vi "SV Get By Measurement Type (voltage) (N Ch).vi"(0 "scaled signals [EU]":waveform(dbl)[](array[waveform])) -> (4 "scaled signals with voltage channels deleted":waveform(dbl)[](array[waveform]), 6 "number of voltage channels":i32, 8 "voltage channels [V]":waveform(dbl)[](array[waveform]))   [LabVIEW 2017]
doc: "Separates data from an array of waveforms based on the type of measurement selected. This VI requires that waveform attributes such as NI_UnitDescription are added by NI DAQmx."
uses:
  <vilib>/addons/_NISVFA/_Shared subVIs/Groups/SV Match Unit.vi
  <vilib>/addons/_NISVFA/_Shared subVIs/Common/sv_Get NI Property Name String.vi
  <vilib>/addons/_NISVFA/_Shared subVIs/Groups/sv_ConcatenateArrayIndicies.vi
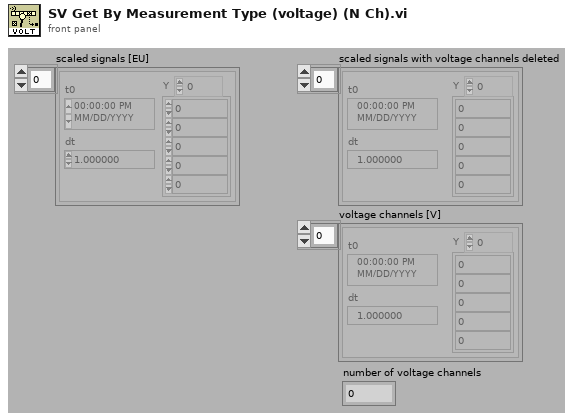
[diagram p1: front panel]
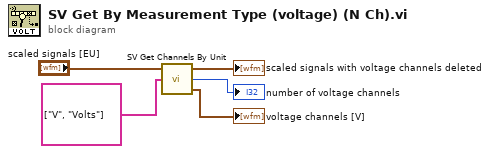
[diagram p0: block diagram]
diagram:
  n1 = call <vilib>:"SV Get Channels By Unit.vi"("units to match"=string[] ["V", "Volts"] ("Units to Match"), "scaled signals [EU]"="scaled signals [EU]") -> ("matching channels [EU]"=→"voltage channels [V]":waveform(dbl)[], "number of matching channels"=→"number of voltage channels":i32, "scaled signals with matching channels deleted"=→"scaled signals with voltage channels deleted":waveform(dbl)[])  [unwired: 1 in]
